vi "DAQmxStrainCONFIG.vi"(8 "error in":errorcluster) -> (0 "error out":errorcluster, 3 "task out":refnum<k21>)   [LabVIEW 2010]
doc: "This VI configures a task.\n\nYour program typically should execute this configuration code only once. To use this code in a loop, use the DAQmx ClearTask VI in the same loop."
uses:
  <vilib>/DAQmx/create/channels.llb/DAQmx Create Channel (AI-Strain-Strain Gage).vi
  <vilib>/DAQmx/configure/timing.llb/DAQmx Timing (Sample Clock).vi
  C:/Program Files/National Instruments/LabVIEW 2010/resource/objmgr/daqmx.rc
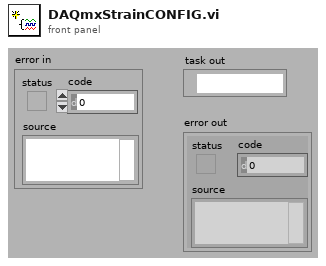
[diagram p1: front panel]
types:
  T1 = cluster{"strain configuration":i32, "lead resistance":dbl, "initial bridge voltage":dbl, "excitation source":i32, "excitation value":dbl}
  T2 = cluster{"gage factor":dbl, "nominal gage resistance":dbl, "poisson ratio":dbl}
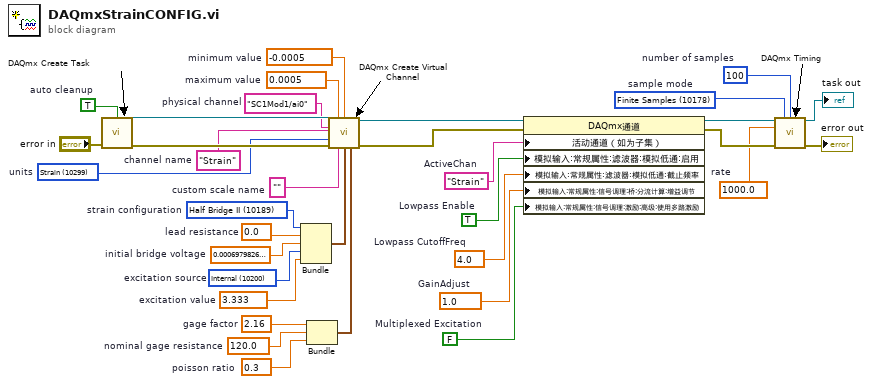
[diagram p0: block diagram]
diagram:
  w1 = 10178 items=["Finite Samples"=10178, "Continuous Samples"=10123]  # sample mode
  w2 = 100  # number of samples
  w3 = 1000.0  # rate
  w6 = FALSE  # Multiplexed Excitation
  w7 = 1.0  # GainAdjust
  w8 = 4.0  # Lowpass CutoffFreq
  w9 = TRUE  # Lowpass Enable
  w12 = "Strain"  # ActiveChan
  w17 = 0.0  # lead resistance
  w20 = 0.3  # poisson ratio
  w16 = 0.0006979826350303459  # initial bridge voltage
  w21 = 120.0  # nominal gage resistance
  w19 = 2.16  # gage factor
  w14 = 3.333  # excitation value
  w15 = 10200 items=["Internal"=10200, "External"=10167, "None"=10230]  # excitation source
  w18 = 10189 items=["Full Bridge I"=10183, "Full Bridge II"=10184, "Full Bridge III"=10185, "Half Bridge I"=10188, "Half Bridge II"=10189, "Quarter Bridge I"=10271, "Quarter Bridge II"=10272]  # strain configuration
  w23 = 10299 items=["Strain"=10299, "From Custom Scale"=10065]  # units
  w24 = "Strain"  # channel name
  w27 = ""  # custom scale name
  w28 = -0.0005  # minimum value
  w29 = 0.0005  # maximum value
  w30 = "SC1Mod1/ai0"  # physical channel
  w31 = TRUE  # auto cleanup
  n1 = call <vilib>:"DAQmx Create Task.vi"("auto cleanup"=w31, "error in"="error in") -> ("task out"=w32:refnum<k21>, "error out"=w33:errorcluster)  [unwired: 12 in]
  n2 = Bundle("strain configuration"=w18, "lead resistance"=w17, "initial bridge voltage"=w16, "excitation source"=w15, "excitation value"=w14) -> (w13:T1)  [unwired: 1 in]
  n3 = Bundle("gage factor"=w19, "nominal gage resistance"=w21, "poisson ratio"=w20) -> (w22:T2)  [unwired: 1 in]
  n4 = call-poly <vilib>:"DAQmx Create Virtual Channel.vi"("task in"=w32, "maximum value"=w29, "minimum value"=w28, "physical channels"=w30, "name to assign"=w24, "units"=w23, "error in"=w33, "custom scale name"=w27, "bridge information"=w13, "strain gage information"=w22) -> ("task out"=w26:refnum<k21>, "error out"=w25:errorcluster)  [unwired: 4 in]
  n5 = property class="DAQmx通道"(reference=w26, error in=w25, "活动通道（如为子集）"=w12, "模拟输入:常规属性:滤波器:模拟低通:启用"=w9, "模拟输入:常规属性:滤波器:模拟低通:截止频率"=w8, "模拟输入:常规属性:信号调理:桥:分流计算:增益调节"=w7, "模拟输入:常规属性:信号调理:激励:高级:使用多路激励"=w6) -> (reference out=w11:refnum<k21>, error out=w10:errorcluster)
  n6 = call-poly <vilib>:"DAQmx Timing.vi"("task/channels in"=w11, "sample mode"=w1, "samples per channel"=w2, "rate"=w3, "error in"=w10) -> ("task out"=→"task out":refnum<k21>, "error out"=→"error out":errorcluster)  [unwired: 9 in]
